vi "解析配置项名与动作.vi"(8 "错误输入":errorcluster) -> (0 "error out":errorcluster, 3 "配置项解析":T1)   [LabVIEW 2017, in "项目开发助手.lvlib" / "模板-配置文件相关.lvlib" / "段-.lvclass"]
uses:
  <vilib>/regexp/Match Regular Expression.xnode
panel:
  out "调用链":string[](array[string])
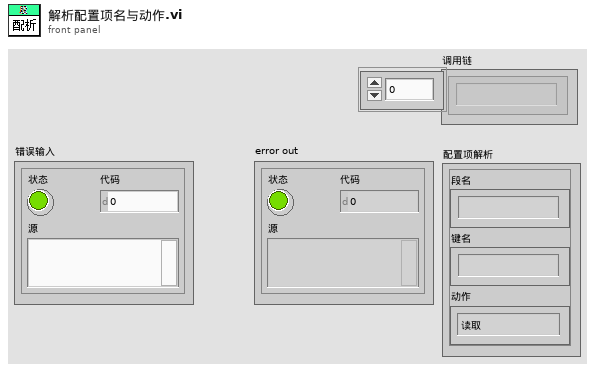
[diagram p1: front panel]
types:
  T1 = typedef "项目开发助手.lvlib/模板-配置文件相关.lvlib/簇-配置文件段键对.ctl" = cluster{"段名":string, "键名":string, "动作":enum16{"读取", "写入"}}
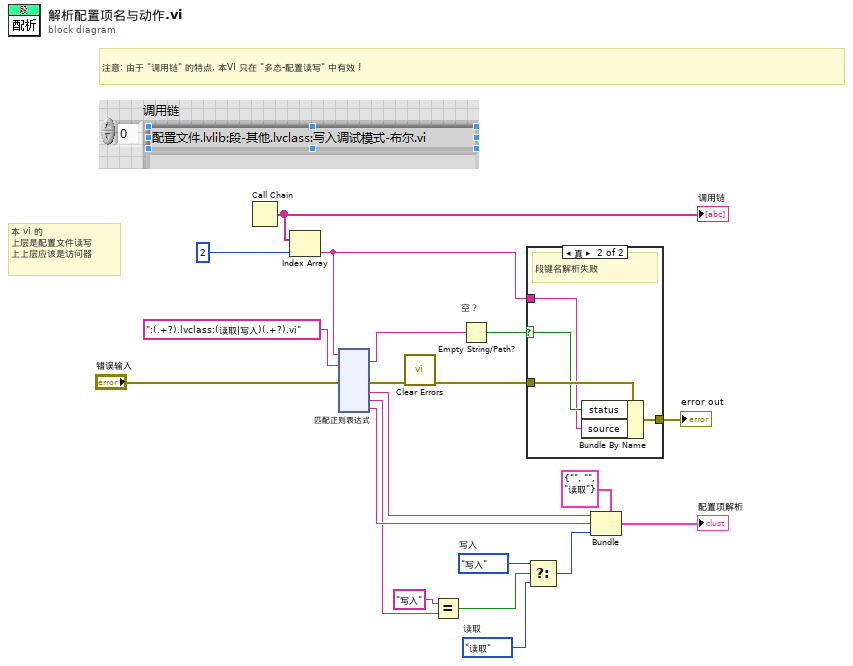
[diagram p0: block diagram]
diagram:
  w5 = enum16{"读取", "写入"}."写入"  # 写入
  w6 = enum16{"读取", "写入"}."读取"  # 读取
  # "注意: 由于 \"调用链\" 的特点, 本VI 只在 \"多态-配置读写\" 中有效 !"
  # "本 vi 的\n上层是配置文件读写\n上上层应该是访问器"
  n1 = Call Chain() -> (call chain=w20:string[])
  "调用链" <- w20
  n2 = Index Array(array=w20, index=2 ("索引")) -> (element=w11:string)
  n3 = xnode "匹配正则表达式"("输入字符串"=w11, "正则表达式"=":(.+?).lvclass:(读取|写入)(.+?).vi" ("输入字符串"), "错误输入"="错误输入") -> ("所有匹配"=w3:string, "错误输出"=w17:errorcluster, "子匹配 1"=w16:string, "子匹配 2"=w9:string, "子匹配 3"=w15:string)  [unwired: 3 in, 3 out]
  n4 = call <vilib>:"Clear Errors.vi"("error in (no error)"=w17) -> ("error out"=w12:errorcluster)  [unwired: 5 in, 1 out]
  n5 = Equal?(x="写入", y=w9) -> (x = y?=w7:bool)
  n6 = Empty String/Path? "空？"(string/path=w3) -> (empty?=w2:bool)
  n7 = case shown="真" w2 {
    selector: w2 -> [_ w24]
    tunnel: w12 -> [w21 w25]
    tunnel: w11 -> [_ w23]
    tunnel: [w21 w22] -> w10
    frame False {
      # "解析段键名成功"
    }
    frame True {
      # "段键名解析失败"
      n8 = Bundle By Name(cluster=w25, "status"=w24, "source"=w23) -> (w22:errorcluster)
    }
  }
  "error out" <- w10
  n9 = Select(t=w5, s=w7, f=w6) -> (s? t:f=w4:enum16{"读取", "写入"})
  n10 = Bundle(cluster=T1 {"段名"="", "键名"="", "动作"=enum."读取"} ("配置项解析"), "段名"=w16, "键名"=w15, "动作"=w4) -> (→"配置项解析":T1)
